vi "U01_15UDPServer.vi"() -> ()   [LabVIEW 2019]
panel:
  out "Sensor 4":bool
  out "Sensor 3":bool
  out "Medidor de flujo":dbl(knob) scale=0.0..10.0
  in  "Generador de Ozono":bool
  out "Slide":u8(slide) scale=0.0..100.0
  out "Pulidor":u8(slide) scale=0.0..100.0
  out "?":u8(slide) scale=0.0..100.0
  out "Meter 2":dbl(knob) scale=0.0..10.0
  out "?":u8(slide) scale=0.0..100.0
  out "Tanque de Agua filtrada":dbl(slide) scale=0.0..10.0
  out "salmuera":dbl(slide) scale=0.0..10.0
  out "filtro arena 3":u8(slide) scale=0.0..100.0
  out "filtro carbon":u8(slide) scale=0.0..100.0
  out "filtro arena":u8(slide) scale=0.0..100.0
  out "?":u8(slide) scale=0.0..100.0
  out "Meter":dbl(knob) scale=0.0..10.0
  out "?":u8(slide) scale=0.0..100.0
  out "Sensor 2":bool
  out "Sensor 1":bool
  out "deposito de agua sin llenar":dbl(slide) scale=0.0..10.0
  out "data out":string
  in  "port":u16
  out "error out":errorcluster
  in  "Tab Control":enum32{"Page 1", "Page 2"}(tab)
  out "?":u8(slide) scale=0.0..100.0
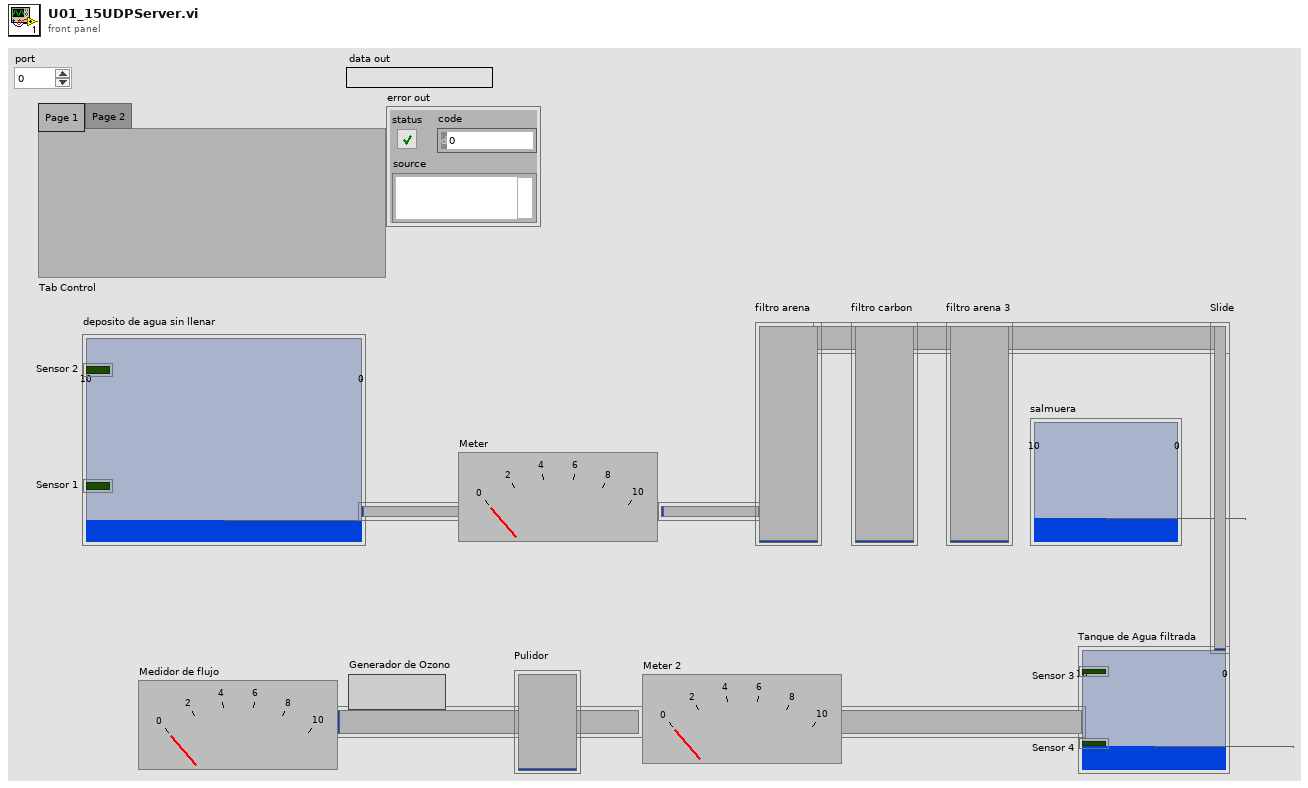
[diagram p1: front panel]
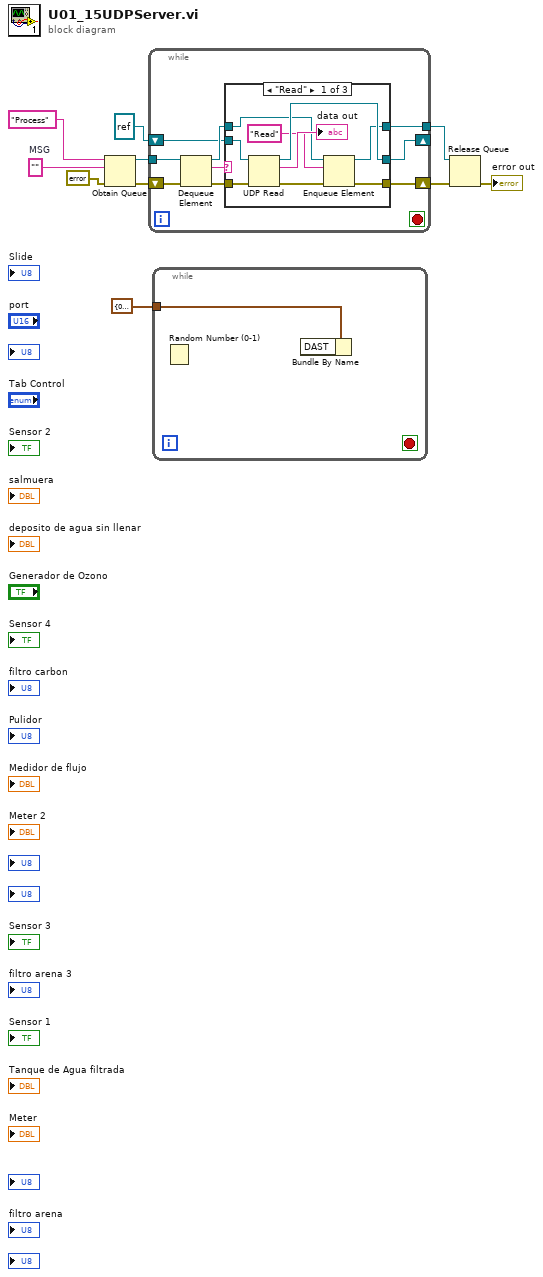
[diagram p0: block diagram]
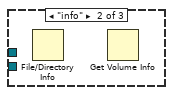
[diagram p2: hidden frame]
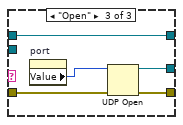
[diagram p3: hidden frame]
diagram:
  w4 = ""  # MSG
  n1 = Obtain Queue(name (unnamed)="Process", element data type=w4, error in (no error)=errorcluster {"status"=FALSE, "code"=0, "source"=""}) -> (queue out=w8:refnum<queue>, error out=w6:errorcluster)  [unwired: 2 in, 1 out]
  n2 = while {
    shift-right: [w14] -> w7
    shift-left: w6 -> [w16]
    tunnel: [w19] -> w9
    tunnel: w8 -> [w18]
    shift-right: [w12] -> _
    shift-left: refnum<k16> refnum ("port") -> [w11]
    stop <- _ stop-if-true
    n3 = Dequeue Element(queue=w18, error in (no error)=w16) -> (queue out=w17:refnum<queue>, element=w15:string, error out=w13:errorcluster)  [unwired: 1 in, 1 out]
    n4 = case shown="\"Read\"" w15 {
      tunnel: w13 -> [w28 _ w32]
      tunnel: [w21 _ w33] -> w19
      tunnel: w17 -> [w22 _ w33]
      tunnel: [w23 _ w31] -> w14
      tunnel: [w26 _ w29] -> w12
      tunnel: w11 -> [w27 _ _]
      frame "Read" {
        n5 = UDP Read(connection ID=w27, 8:w28) -> (data out=→"data out":string, error out=w24:errorcluster, 3:w26:refnum<k16>)  [unwired: 2 in, 2 out]
        n6 = Enqueue Element(queue=w22, element="Read", error in (no error)=w24) -> (queue out=w21:refnum<queue>, error out=w23:errorcluster)  [unwired: 1 in, 1 out]
      }
      frame "info" {
        n7 = File/Directory Info() -> ()  [unwired: 2 in, 7 out]
        n8 = Get Volume Info() -> ()  [unwired: 2 in, 6 out]
      }
      frame "Open" {
        n9 = property on="port" class="DigNum (strict)"() -> ("Value"=w30:u16)  [unwired: 2 in, 2 out]
        n10 = UDP Open(8:w32, 11:w30) -> (port=w29:refnum<k16>, 0:w31:errorcluster)  [unwired: 3 in, 1 out]
      }
    }
  }
  n11 = while {
    tunnel: cluster{"DAST":dbl, "SMU":dbl, "AT":dbl} {"DAST"=0.0, "SMU"=0.0, "AT"=0.0} -> [w34]
    stop <- _ stop-if-true
    n12 = Random Number (0-1)() -> ()  [unwired: 1 out]
    n13 = Bundle By Name(cluster=w34) -> ()  [unwired: 1 in, 1 out]
  }
  n14 = Release Queue(queue=w9, error in (no error)=w7) -> (error out=→"error out":errorcluster)  [unwired: 1 in, 2 out]
